vi "Template Get by sxTemplateId.vi"(8 "error in (no error)":errorcluster, 10 "sxTemplateId (\"\")":string, 11 "Connection Refnum":T2) -> (0 "error out":errorcluster, 1 "Parameters":T1, 2 "Template Record":T3, 3 "Connection Refnum":T2, 4 "Data Present":bool, 6 "ini file Missing":bool)   [LabVIEW 2011]
uses:
  Template Record.ctl
  Summitek EXT/ODBC/SQL Controls/Connection Refnum.ctl
  ITK EXT/utils/keyedarr.llb/Keyed Array.ctl
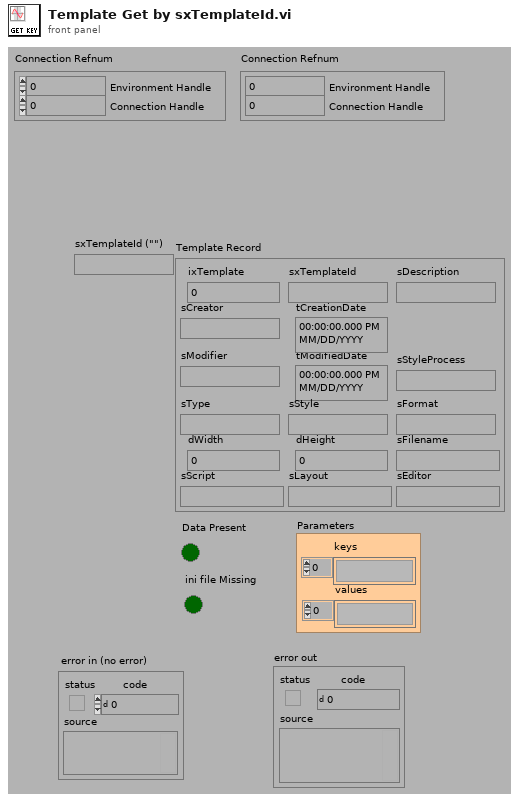
[diagram p1: front panel]
types:
  T1 = typedef "Keyed Array.ctl" = cluster{"keys":string[], "values":string[]}
  T2 = typedef "Connection Refnum.ctl" = cluster{"Environment Handle":i32, "Connection Handle":i32}
  T3 = typedef "Template Record.ctl" = cluster{"ixTemplate":i32, "sxTemplateId":string, "sDescription":string, "sCreator":string, "tCreationDate":timestamp, "sModifier":string, "tModifiedDate":timestamp, "sType":string, "sStyle":string, "sFormat":string, "dWidth":dbl, "dHeight":dbl, "sFilename":string, "sScript":string, "sLayout":string, "sEditor":string, "sStyleProcess":string}
  T4 = typedef "Statement Refnum.ctl" = cluster{"Statement Handle":i32, "Parameter Number":u16}
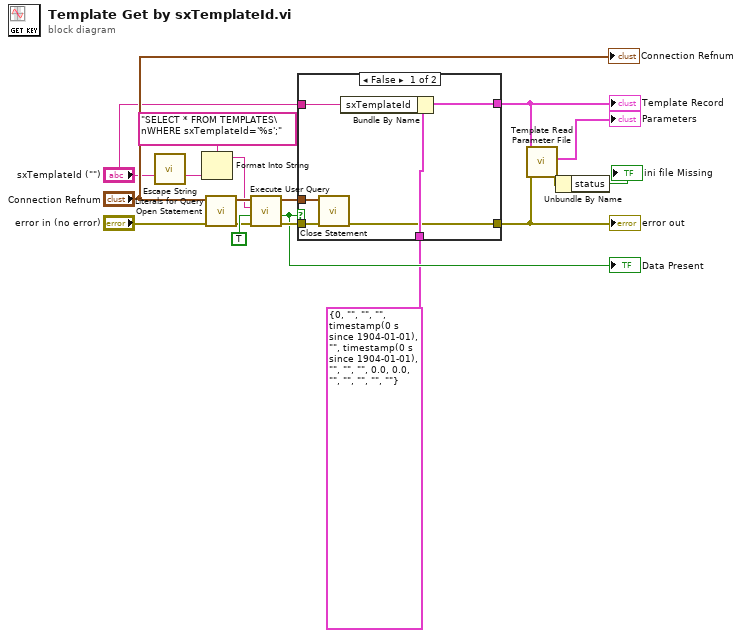
[diagram p0: block diagram]
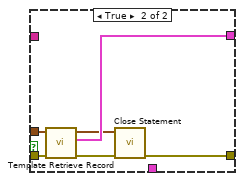
[diagram p2: hidden frame]
diagram:
  n1 = call "Escape String Literals for Query.vi"("String"="sxTemplateId (\"\")") -> ("escaped String"=w9:string)  [unwired: 1 in, 13 out]
  n2 = Format Into String(format string="SELECT * FROM TEMPLATES\nWHERE sxTemplateId='%s';" ("User Query"), w9) -> (resulting string=w12:string)  [unwired: 2 in, 1 out]
  n3 = call "Open Statement.vi"("error in (no error)"="error in (no error)", "Connection Refnum"="Connection Refnum") -> ("error out"=w13:errorcluster, "Statement Refnum"=w14:T4)  [unwired: 4 out]
  n4 = call "Execute User Query.vi"("error in (no error)"=w13, "Return Data? (f)"=TRUE, "User Query"=w12, "Statement Refnum"=w14) -> ("error out"=w18:errorcluster, "Data Present?"=w8:bool, "Statement Refnum"=w17:T4)  [unwired: 1 out]
  "Data Present" <- w8
  n5 = case shown="False" w8 {
    tunnel: w18 -> [w20 w29]
    tunnel: w17 -> [w21 w30]
    tunnel: [w19 w25] -> w3
    tunnel: [w24 w28] -> w4
    tunnel: T3 {"ixTemplate"=0, "sxTemplateId"="", "sDescription"="", "sCreator"="", "tCreationDate"=timestamp(0 s since 1904-01-01), "sModifier"="", "tModifiedDate"=timestamp(0 s since 1904-01-01), "sType"="", "sStyle"="", "sFormat"="", "dWidth"=0.0, "dHeight"=0.0, "sFilename"="", "sScript"="", "sLayout"="", "sEditor"="", "sStyleProcess"=""} ("Template Record") -> [w23 _]
    tunnel: "sxTemplateId (\"\")" -> [w22 _]
    frame False {
      n6 = call "Close Statement.vi"("error in (no error)"=w20, "Statement Refnum"=w21) -> ("error out"=w19:errorcluster)  [unwired: 5 out]
      n7 = Bundle By Name(cluster=w23, "sxTemplateId"=w22) -> (w24:T3)
    }
    frame True {
      n8 = call "Template Retrieve Record.vi"("error in (no error)"=w29, "Statement Refnum"=w30) -> ("error out"=w27:errorcluster, "Template Record"=w28:T3, "Statement Refnum"=w26:T4)  [unwired: 7 out]
      n9 = call "Close Statement.vi"("error in (no error)"=w27, "Statement Refnum"=w26) -> ("error out"=w25:errorcluster)  [unwired: 5 out]
    }
  }
  "error out" <- w3
  "Template Record" <- w4
  n10 = call "Template Read Parameter File.vi"("error in (no error)"=w3, "Template Record"=w4) -> ("error out"=w2:errorcluster, "Parameters"=→"Parameters":T1)  [unwired: 1 in, 7 out]
  n11 = Unbundle By Name(w2) -> ("status"=→"ini file Missing":bool)
  "Connection Refnum" <- "Connection Refnum"
